vi "XY Dialog.vi"(8 "error in (no error)":errorcluster, 10 "Waveform Graph Data in":T1={"Custom Data"=variant, "EventRegs"={"SystemChange"=refnum, "WorkspaceState"=refnum, "Graph"=refnum, "Wks&Dialog&Periodic"=refnum}, "References"={"X.Scale.Auto"=refnum, "Y.Scale.Auto"=refnum, "X.Scale.Once"=refnum, "Y.Scale.Once"=refnum, "LegendVis"=refnum, "Graph"=refnum}, "Persistent Data"={"Label"="", "Graph Props"={"Plots"=[], "Legend:Number of Rows"=0, "Scale Properties"={"X.Auto"=FALSE, "X.Min"=0.0, "X.Max"=0.0, "X.IgnoreTS"=FALSE, "X.Precision"=0, "X.Label:"="", "X.LabelVis"=FALSE, "X.DefLabel"=FALSE, "Y.Auto"=FALSE, "Y.Min"=0.0, "Y.Max"=0.0, "Y.Format"=0, "Y.Precision:"=0, "Y.Label:"="", "Y.LabelVis"=FALSE, "Y.DefLabel"=FALSE, "X.Format"=0}, "Legend:Visible"=TRUE, "BgColor"=0, "Last Plot Width"=0, "Resize"=FALSE}, "UDP Data"={"Decimation"=0, "UDP Buffer Size"=0, "History Length"=0.0, "Update Rate"=enum."15 Hz", "Channel Paths"=[], "Channel Names"=[]}}, "System"={"To Workspace"=refnum, "From Workspace"=refnum, "NIVS helper"=refnum, "Gtwy"="", "Root"=refnum, "Workspace"=refnum, "SystemStateRefs"={"CustDatRef"=refnum, "EvtRef"=refnum}, "Connected?"=FALSE, "FromDialog"=refnum, "ErrFlag"=FALSE, "New"=FALSE, "ErrState"="", "Save"=FALSE, "Hold"=FALSE, "Periodic"=refnum, "ToDialog"=refnum, "DialogEventReg"=refnum, "UseSavedWidth"=FALSE, "TreeBrowserEventReg"=refnum, "UDPChannelStreamSession"=refnum, "Valid Channels?"=FALSE, "Update Graph"=refnum, "UDP Queue"=refnum, "Graph Update Queue"=refnum}, "GraphData"=[], "UDP Stream Active?"=FALSE} {"Persistent Data"."Graph Props"."Scale Properties"."X.Format" items=["Decimal", "Scientific", "Engineering", "Binary", "Octal", "Hexadecimal", "Relative Time", "Time and Date", "SI", "Automatic"]; "Persistent Data"."Graph Props"."Scale Properties"."Y.Precision:" items=["0", "1", "2", "3", "4", "5", "6", "7"]; "Persistent Data"."Graph Props"."Scale Properties"."Y.Format" items=["Decimal", "Scientific", "Engineering", "Binary", "Octal", "Hexadecimal", "Relative Time", "Time and Date", "SI", "Automatic"]; "Persistent Data"."Graph Props"."Scale Properties"."X.Precision" items=["0", "1", "2", "3", "4", "5", "6", "7"]}) -> ()   [LabVIEW 2013, in "Workspace MultiY Graph.lvlib"]
uses:
  Workspace MultiY Graph.lvlib
  XY Scale Precision.ctl
  XY Scale Format.ctl
  XY Top level workspace graph data.ctl
  <vilib>/NI Veristand/Execution/Workspace/SystemStateRegEventRef.ctl
  <vilib>/NI Veristand/Display Template Support/Display Template Support.llb/enum_Display Template Handler Minimal To Widget Msg.ctl
  XY Dialog Msg to Control.ctl
  XY Dialog Msg Type.ctl
  XY Persistent Data.ctl
  XY Graph Properties.ctl
  XY Plot Properties.ctl
  XY Scale Properties.ctl
  UDP Data.ctl
  Update Rate.ctl
  XY References.ctl
  <vilib>/NI Veristand/Display Template Support/Display Template Support.llb/enum_Display Template Handler Minimal To Workspace.ctl
  NationalInstruments.VeriStand.SystemStorage
  <vilib>/NI Veristand/Execution/Workspace/WorkspaceAPI.ctl
  NationalInstruments.VeriStand.ClientAPI
  <vilib>/NI Veristand/Execution/Workspace/SystemStateEventRef.ctl
  XY Control Msg to Dialog.ctl
  <vilib>/NI Veristand/UI Controls/Tree and Alias Browser/Net Event Data Ref.ctl
  <vilib>/NI Veristand/UI Controls/Tree and Alias Browser/Net Event Data.ctl
  <vilib>/NI Veristand/UI Controls/Tree and Alias Browser/Net Event.ctl
  <vilib>/NI Veristand/Execution/Workspace/UDPChannelStreamSession.ctl
  UDP Queue Data.ctl
  UDP Action State.ctl
  Graph Update Queue Data.ctl
  Graph Update Action State.ctl
  NationalInstruments.VeriStand.SystemStorageUI
  XY Top level dialog data.ctl
  XY Dialog References.ctl
  Dlg Symbol.ctl
  <vilib>/NI Veristand/Execution/Workspace/NI_VS Workspace ExecutionAPI.lvlib
  <vilib>/NI Veristand/UI Controls/Tree and Alias Browser/NI_VS UI Tree Alias Browser.lvlib
  Alert Dialogs.lvlib
panel:
  in  "Cancel":bool
  in  "OK":bool
  in  "Delete":bool
  in  "Tab Control":enum32{"General", "Format & Precision"}(tab)
  in  "Y Channel":i32[](listbox)
  in  "Y Previous":bool
  in  "Y Next":bool
  in  "Tree Browser":refnum<k24>(container)
  in  "X Channel":i32[](listbox)
  in  "X Previous":bool
  in  "X Next":bool
  in  "Resize":bool
  in  "Update Rate:":T11
  in  "History Length:":dbl=0.5 min=0.5 max=3600.0 step=0.5
  in  "UDP Buffer Size:":u32=8192 min=8192 max=65536 step=1
  in  "Decimation:":i32=1 min=1 max=1000000 step=1
  in  "Plot Area Background Color":u32(colorbox)
  in  "Graph Title":string="Waveform Graph"
  in  "X.Format":T9 caption="Format:" items=["Decimal", "Scientific", "Engineering", "Binary", "Octal", "Hexadecimal", "Relative Time", "Time and Date", "SI", "Automatic"]
  in  "X.Min":dbl caption="Minimum:"
  in  "X.Max":dbl caption="Maximum:"
  in  "X.Precision":T8 caption="Precision:" items=["0", "1", "2", "3", "4", "5", "6", "7"]
  in  "Y.Precision":T8 caption="Precision:" items=["0", "1", "2", "3", "4", "5", "6", "7"]
  in  "Y.Format":T9 caption="Format:" items=["Decimal", "Scientific", "Engineering", "Binary", "Octal", "Hexadecimal", "Relative Time", "Time and Date", "SI", "Automatic"]
  in  "X.Label.Default":bool caption="Use Default Label?"
  in  "X.Label.Visible":bool caption="Label Visible?"
  in  "X.Label":string caption="Label:"
  in  "Y.Label.Default":bool caption="Use Default Label?"
  in  "Y.Label.Visible":bool caption="Label Visible?"
  in  "Y.Label":string caption="Label:"
  in  "X.Autoscale":bool caption="Autoscale?"
  in  "Y.Autoscale":bool caption="Autoscale?"
  in  "Y.Min":dbl caption="Minimum:"
  in  "Y.Max":dbl caption="Maximum:"
  # "X Scale"
  # "Y Scale"
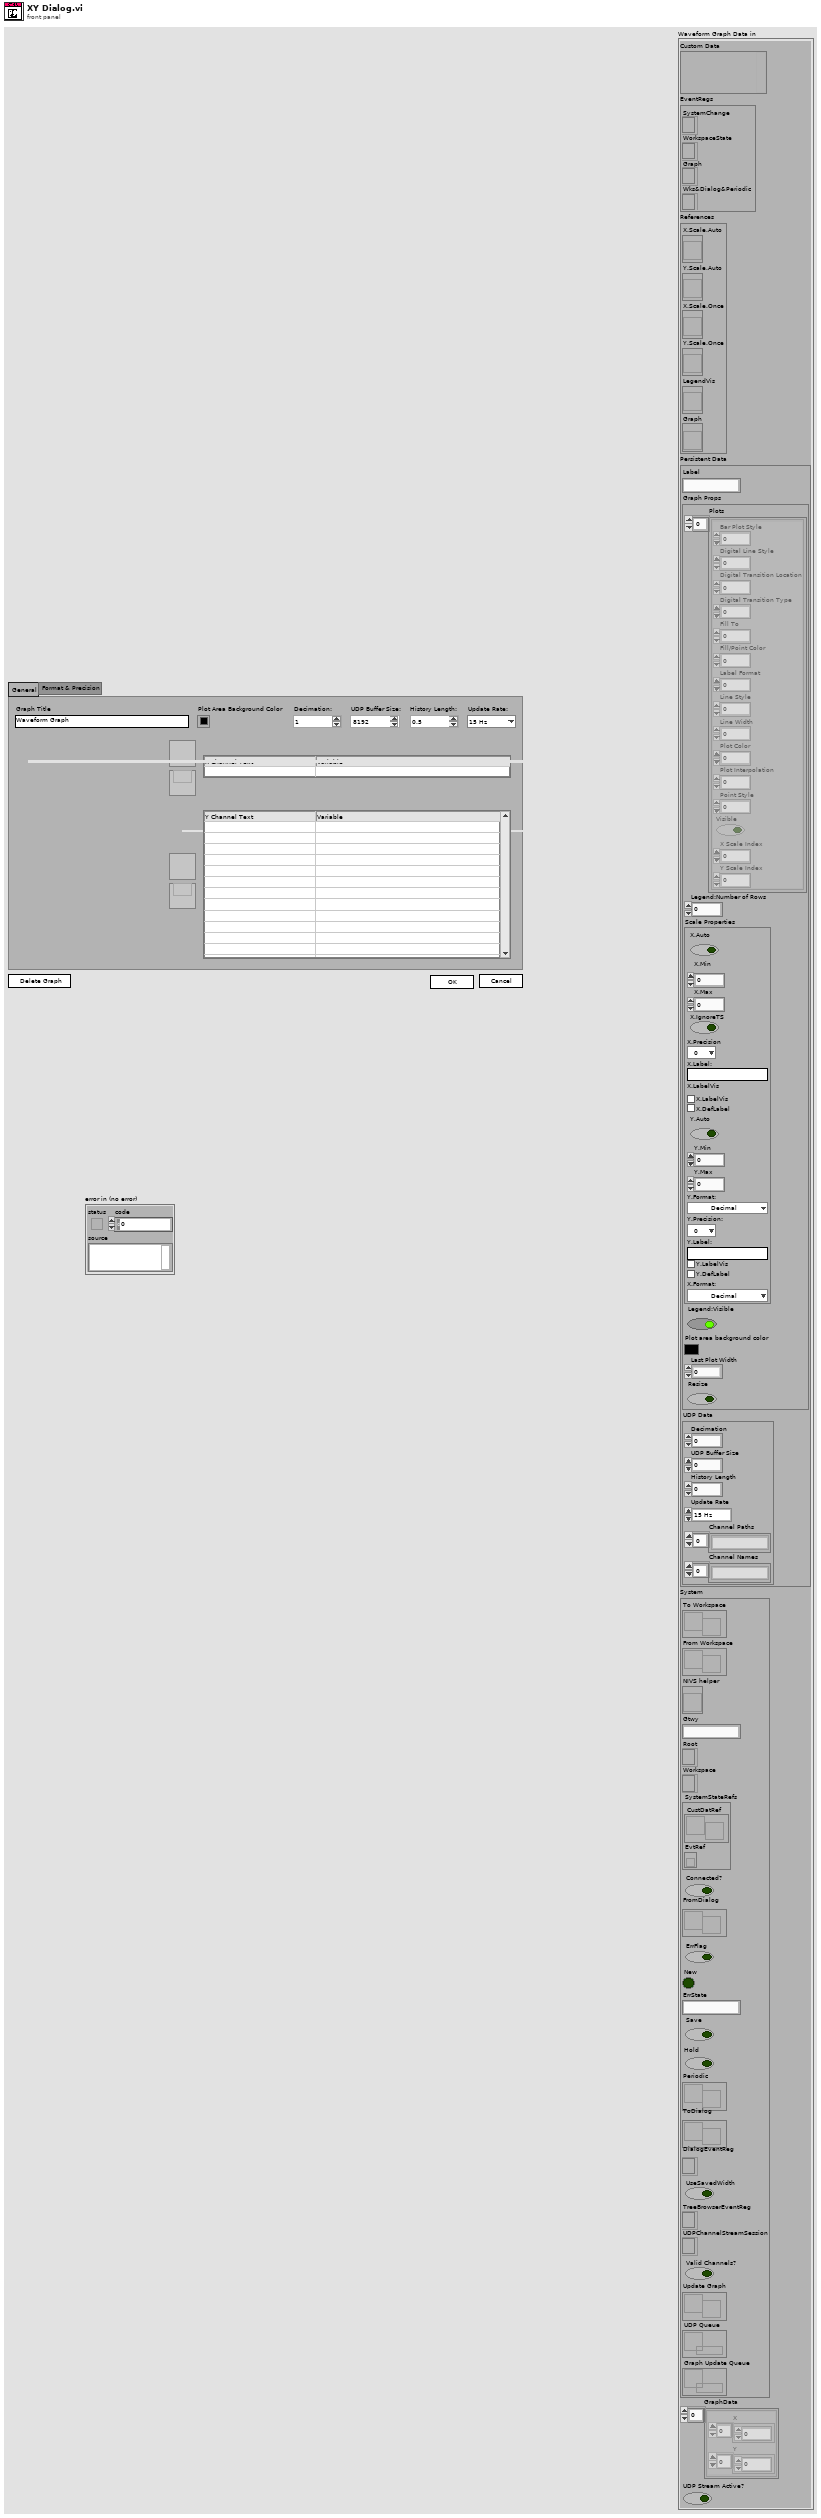
[diagram p1: front panel]
types:
  T1 = typedef "Workspace MultiY Graph.lvlib/XY Top level workspace graph data.ctl" = cluster{"Custom Data":variant, "EventRegs":cluster{"SystemChange":T2, "WorkspaceState":refnum<event-registration>, "Graph":refnum<event-registration>, "Wks&Dialog&Periodic":refnum<event-registration>}, "References":T3, "Persistent Data":T4, "System":cluster{"To Workspace":refnum<user-event>, "From Workspace":refnum<user-event>, "NIVS helper":refnum<vi>, "Gtwy":string, "Root":refnum<k24>, "Workspace":T12, "SystemStateRefs":T13, "Connected?":bool, "FromDialog":refnum<user-event>, "ErrFlag":bool, "New":bool, "ErrState":string, "Save":bool, "Hold":bool, "Periodic":refnum<user-event>, "ToDialog":refnum<user-event>, "DialogEventReg":refnum<event-registration>, "UseSavedWidth":bool, "TreeBrowserEventReg":refnum<event-registration>, "UDPChannelStreamSession":T14, "Valid Channels?":bool, "Update Graph":refnum<user-event>, "UDP Queue":refnum<queue>, "Graph Update Queue":refnum<queue>}, "GraphData":cluster{"X":dbl[], "Y":dbl[]}[], "UDP Stream Active?":bool}
  T2 = typedef "NI_VS Workspace ExecutionAPI.lvlib/SystemStateRegEventRef.ctl" = refnum<event-registration>
  T3 = typedef "Workspace MultiY Graph.lvlib/XY References.ctl" = cluster{"X.Scale.Auto":refnum<vi>, "Y.Scale.Auto":refnum<vi>, "X.Scale.Once":refnum<vi>, "Y.Scale.Once":refnum<vi>, "LegendVis":refnum<vi>, "Graph":refnum<vi>}
  T4 = typedef "Workspace MultiY Graph.lvlib/XY Persistent Data.ctl" = cluster{"Label":string, "Graph Props":T5, "UDP Data":T10}
  T5 = typedef "Workspace MultiY Graph.lvlib/XY Graph Properties.ctl" = cluster{"Plots":T6[], "Legend:Number of Rows":u32, "Scale Properties":T7, "Legend:Visible":bool, "BgColor":u32, "Last Plot Width":u32, "Resize":bool}
  T6 = typedef "Workspace MultiY Graph.lvlib/XY Plot Properties.ctl" = cluster{"Bar Plot Style":u8, "Digital Line Style":u8, "Digital Transition Location":u8, "Digital Transition Type":u8, "Fill To":i16, "Fill/Point Color":u32, "Label Format":u8, "Line Style":u8, "Line Width":u8, "Plot Color":u32, "Plot Interpolation":u8, "Point Style":u8, "Visible":bool, "X Scale Index":u32, "Y Scale Index":u32}
  T7 = typedef "Workspace MultiY Graph.lvlib/XY Scale Properties.ctl" = cluster{"X.Auto":bool, "X.Min":dbl, "X.Max":dbl, "X.IgnoreTS":bool, "X.Precision":T8, "X.Label:":string, "X.LabelVis":bool, "X.DefLabel":bool, "Y.Auto":bool, "Y.Min":dbl, "Y.Max":dbl, "Y.Format":T9, "Y.Precision:":T8, "Y.Label:":string, "Y.LabelVis":bool, "Y.DefLabel":bool, "X.Format":T9}
  T8 = typedef "Workspace MultiY Graph.lvlib/XY Scale Precision.ctl" = u8
  T9 = typedef "Workspace MultiY Graph.lvlib/XY Scale Format.ctl" = u8
  T10 = typedef "Workspace MultiY Graph.lvlib/UDP Data.ctl" = cluster{"Decimation":i32, "UDP Buffer Size":u32, "History Length":dbl, "Update Rate":T11, "Channel Paths":string[], "Channel Names":string[]}
  T11 = typedef "Workspace MultiY Graph.lvlib/Update Rate.ctl" = enum8{"15 Hz", "10 Hz", "5 Hz", "4 Hz", "3 Hz", "2 Hz", "1 Hz", "0.5 Hz"}
  T12 = typedef "NI_VS Workspace ExecutionAPI.lvlib/WorkspaceAPI.ctl" = refnum<k24>
  T13 = typedef "NI_VS Workspace ExecutionAPI.lvlib/SystemStateEventRef.ctl" = cluster{"CustDatRef":refnum<user-event>, "EvtRef":refnum<k27>}
  T14 = typedef "NI_VS Workspace ExecutionAPI.lvlib/UDPChannelStreamSession.ctl" = refnum<k24>
  T15 = typedef "Workspace MultiY Graph.lvlib/XY Top level dialog data.ctl" = cluster{"GraphData":T1, "References":T16, "Tree Selected Paths":string[][], "SelectedIdx":i32, "dts":dbl[], "X Selected Paths":string[][], "Y Selected Paths":string[][]}
  T16 = typedef "Workspace MultiY Graph.lvlib/XY Dialog References.ctl" = cluster{"BgColor":refnum<vi>, "Title":refnum<vi>, "Waveforms":refnum<vi>, "PointsPerPixel":refnum<vi>, "Low":refnum<vi>, "High":refnum<vi>, "History":refnum<vi>, "N":refnum<vi>, "M":refnum<vi>, "IgnTimeStamp":refnum<vi>, "X.Precision":refnum<vi>, "X.Label":refnum<vi>, "X.Label.Default":refnum<vi>, "X.Label.Visible":refnum<vi>, "X.Autoscale":refnum<vi>, "X.Max":refnum<vi>, "X.Min":refnum<vi>, "Y.Format":refnum<vi>, "Y.Precision":refnum<vi>, "Y.Label":refnum<vi>, "Y.Label.Default":refnum<vi>, "Y.Label.Visible":refnum<vi>, "Y.Autoscale":refnum<vi>, "Y.Max":refnum<vi>, "Y.Min":refnum<vi>, "rate":refnum<vi>, "path":refnum<vi>, "Alias TreeBrowser":refnum<vi>, "Y Channel Listbox":refnum<vi>, "X Channel Listbox":refnum<vi>, "X.Format":refnum<vi>, "X Next":refnum<vi>, "Y Next":refnum<vi>, "X Previous":refnum<vi>, "Y Previous":refnum<vi>, "Decimation":refnum<vi>, "History Length":refnum<vi>, "UDP Buffer Size":refnum<vi>}
  T17 = typedef "Workspace MultiY Graph.lvlib/Alert Dialogs.lvlib/Dlg Symbol.ctl" = enum16{"Information", "Help", "Warning", "Error"}
  T18 = enum8{"Enabled", "Disabled", "Disabled and Grayed Out"}
  T19 = typedef "Workspace MultiY Graph.lvlib/XY Dialog Msg Type.ctl" = enum16{"Update", "Delete"}
  T20 = typedef "Workspace MultiY Graph.lvlib/XY Dialog Msg to Control.ctl" = cluster{"DialogMsgType":T19, "Persistent Data":T4}
  T21 = cluster{"TreeBrowserEventReg":refnum<event-registration>, "DialogEventReg":refnum<event-registration>}
  T22 = typedef "Workspace MultiY Graph.lvlib/XY Control Msg to Dialog.ctl" = enum16{"Stop", "Connecting", "Disconnecting"}
  T23 = typedef "Workspace MultiY Graph.lvlib/Alert Dialogs.lvlib/Dlg Button.ctl" = enum16{"Left Button", "Center Button", "Right Button", "Window Close"}
  T24 = typedef "NI_VS UI Tree Alias Browser.lvlib/Net Event.ctl" = enum16{"SelectedItem", "DblClick"}
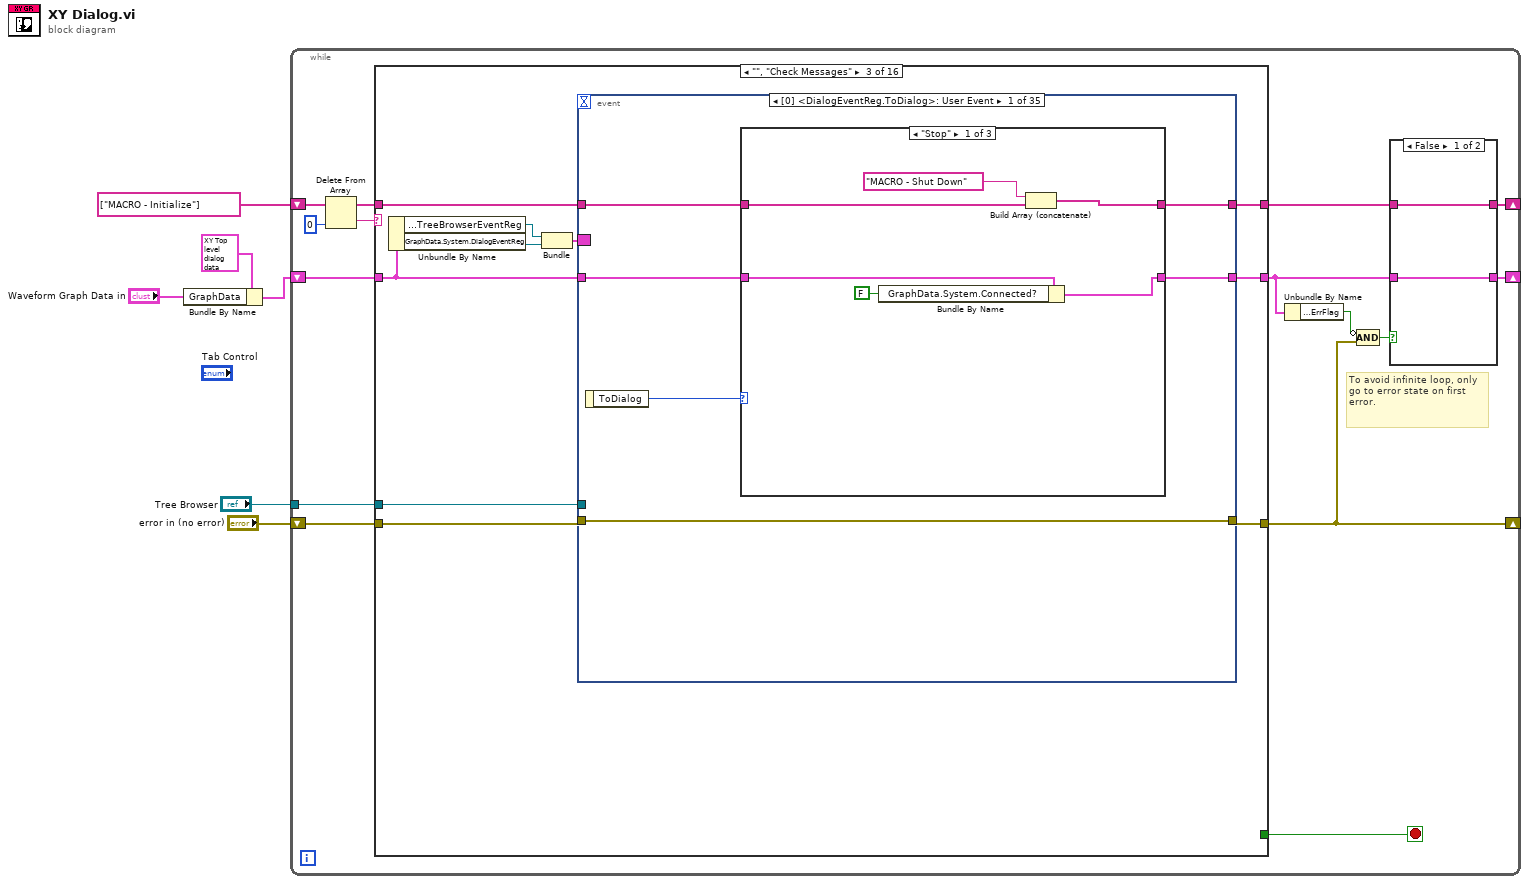
[diagram p0: block diagram]
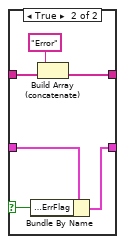
[diagram p2: hidden frame]
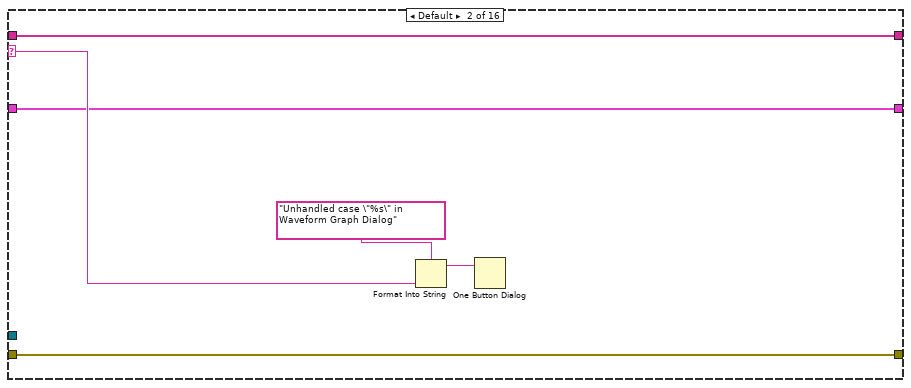
[diagram p4: hidden frame]
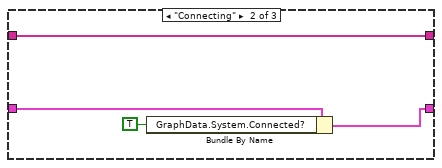
[diagram p5: hidden frame]
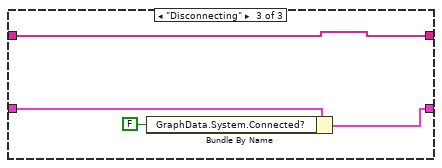
[diagram p6: hidden frame]
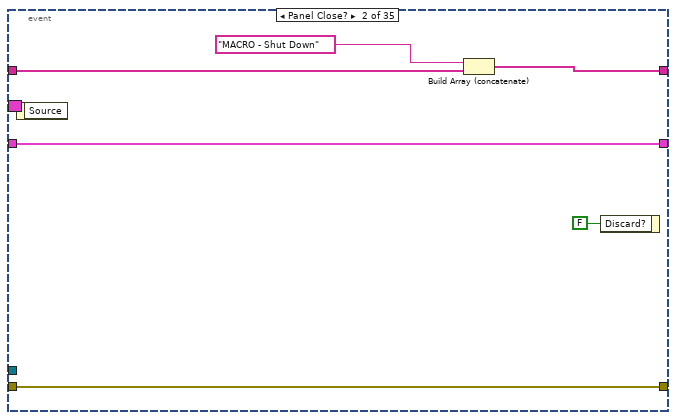
[diagram p7: hidden frame]
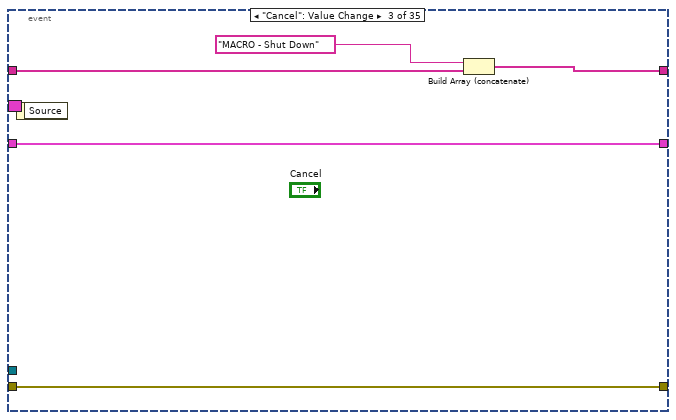
[diagram p8: hidden frame]
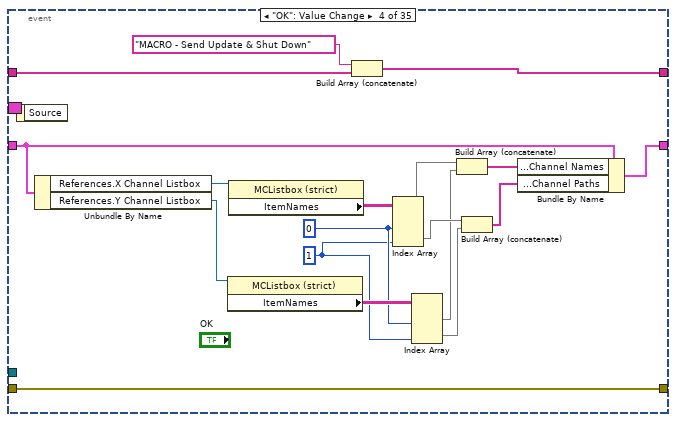
[diagram p9: hidden frame]
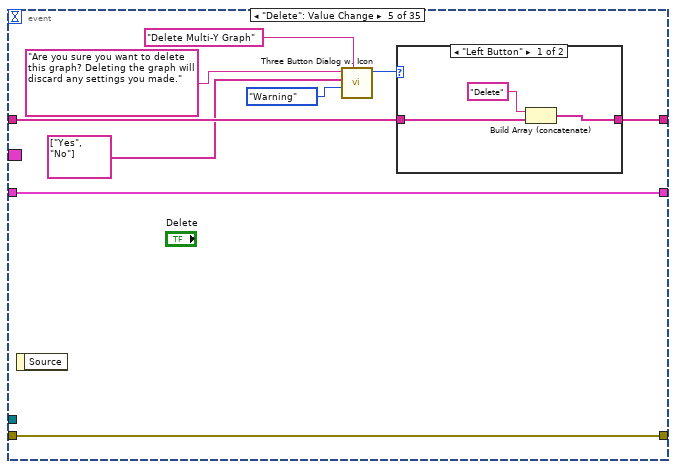
[diagram p10: hidden frame]
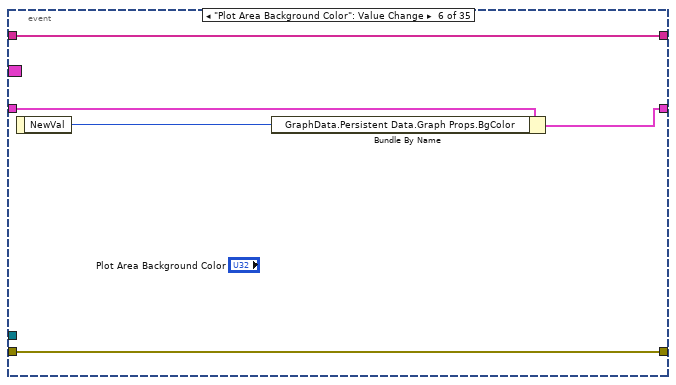
[diagram p12: hidden frame]
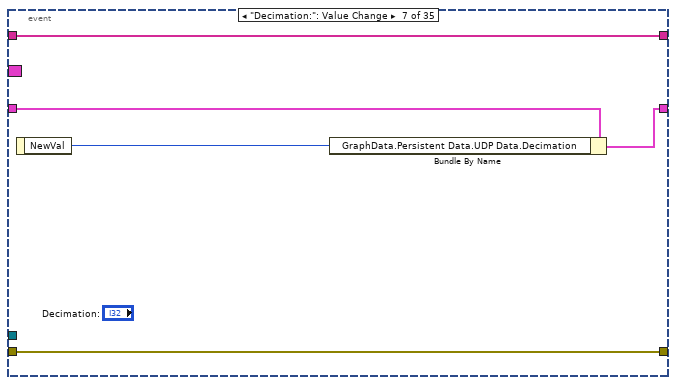
[diagram p13: hidden frame]
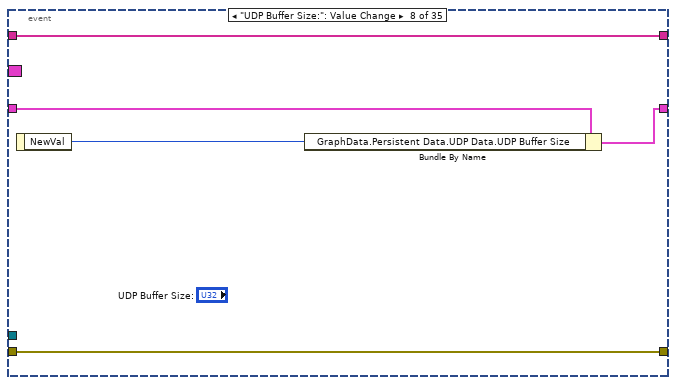
[diagram p14: hidden frame]
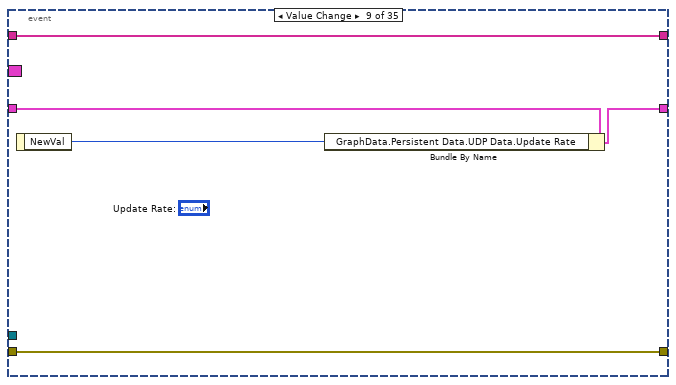
[diagram p15: hidden frame]
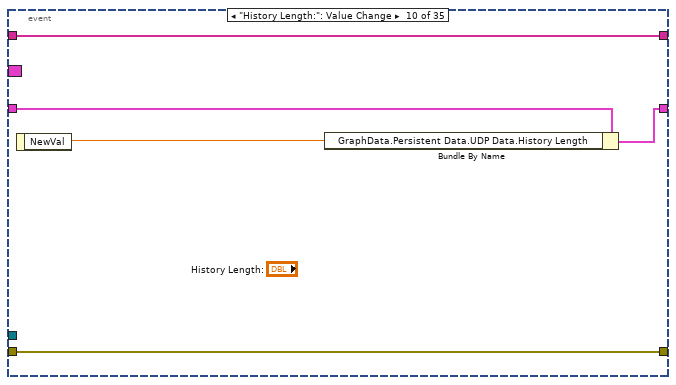
[diagram p16: hidden frame]
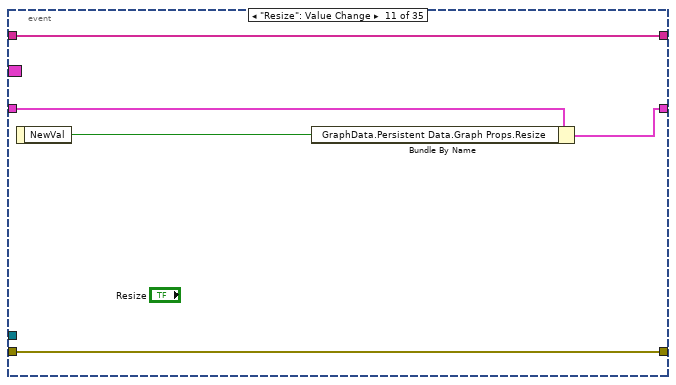
[diagram p17: hidden frame]
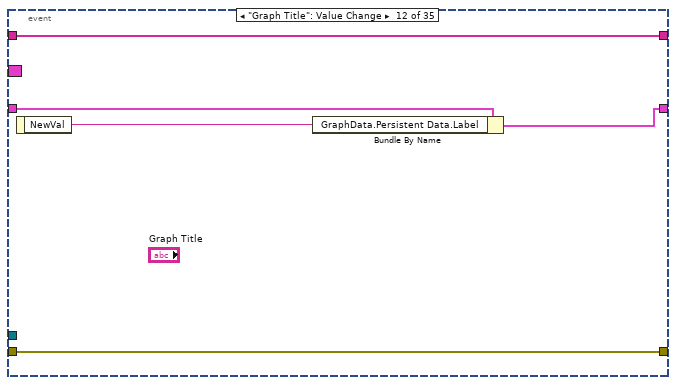
[diagram p18: hidden frame]
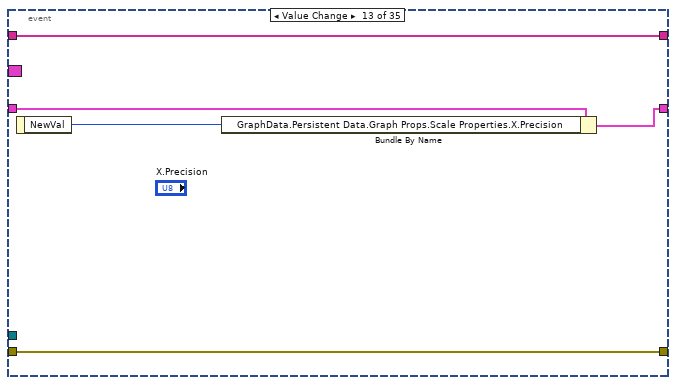
[diagram p19: hidden frame]
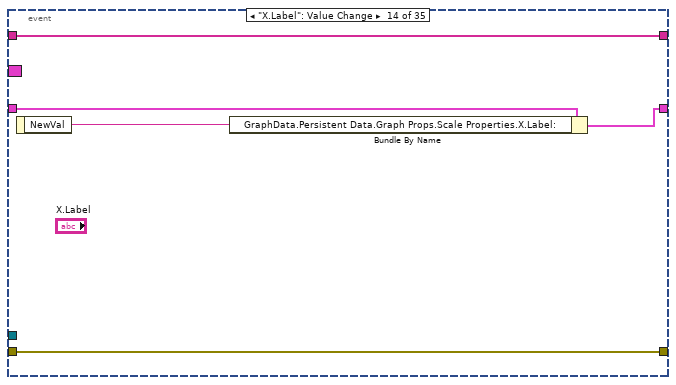
[diagram p20: hidden frame]
diagram:
  n1 = Bundle By Name(cluster=T15 {"GraphData"={"Custom Data"=variant, "EventRegs"={"SystemChange"=refnum, "WorkspaceState"=refnum, "Graph"=refnum, "Wks&Dialog&Periodic"=refnum}, "References"={"X.Scale.Auto"=refnum, "Y.Scale.Auto"=refnum, "X.Scale.Once"=refnum, "Y.Scale.Once"=refnum, "LegendVis"=refnum, "Graph"=refnum}, "Persistent Data"={"Label"="", "Graph Props"={"Plots"=[], "Legend:Number of Rows"=0, "Scale Properties"={"X.Auto"=FALSE, "X.Min"=0.0, "X.Max"=0.0, "X.IgnoreTS"=FALSE, "X.Precision"=0, "X.Label:"="", "X.LabelVis"=FALSE, "X.DefLabel"=FALSE, "Y.Auto"=FALSE, "Y.Min"=0.0, "Y.Max"=0.0, "Y.Format"=0, "Y.Precision:"=0, "Y.Label:"="", "Y.LabelVis"=FALSE, "Y.DefLabel"=FALSE, "X.Format"=0}, "Legend:Visible"=FALSE, "BgColor"=0, "Last Plot Width"=0, "Resize"=FALSE}, "UDP Data"={"Decimation"=0, "UDP Buffer Size"=0, "History Length"=0.0, "Update Rate"=enum."15 Hz", "Channel Paths"=[], "Channel Names"=[]}}, "System"={"To Workspace"=refnum, "From Workspace"=refnum, "NIVS helper"=refnum, "Gtwy"="", "Root"=refnum, "Workspace"=refnum, "SystemStateRefs"={"CustDatRef"=refnum, "EvtRef"=refnum}, "Connected?"=FALSE, "FromDialog"=refnum, "ErrFlag"=FALSE, "New"=FALSE, "ErrState"="", "Save"=FALSE, "Hold"=FALSE, "Periodic"=refnum, "ToDialog"=refnum, "DialogEventReg"=refnum, "UseSavedWidth"=FALSE, "TreeBrowserEventReg"=refnum, "UDPChannelStreamSession"=refnum, "Valid Channels?"=FALSE, "Update Graph"=refnum, "UDP Queue"=refnum, "Graph Update Queue"=refnum}, "GraphData"=[], "UDP Stream Active?"=FALSE}, "References"={"BgColor"=refnum, "Title"=refnum, "Waveforms"=refnum, "PointsPerPixel"=refnum, "Low"=refnum, "High"=refnum, "History"=refnum, "N"=refnum, "M"=refnum, "IgnTimeStamp"=refnum, "X.Precision"=refnum, "X.Label"=refnum, "X.Label.Default"=refnum, "X.Label.Visible"=refnum, "X.Autoscale"=refnum, "X.Max"=refnum, "X.Min"=refnum, "Y.Format"=refnum, "Y.Precision"=refnum, "Y.Label"=refnum, "Y.Label.Default"=refnum, "Y.Label.Visible"=refnum, "Y.Autoscale"=refnum, "Y.Max"=refnum, "Y.Min"=refnum, "rate"=refnum, "path"=refnum, "Alias TreeBrowser"=refnum, "Y Channel Listbox"=refnum, "X Channel Listbox"=refnum, "X.Format"=refnum, "X Next"=refnum, "Y Next"=refnum, "X Previous"=refnum, "Y Previous"=refnum, "Decimation"=refnum, "History Length"=refnum, "UDP Buffer Size"=refnum}, "Tree Selected Paths"=[], "SelectedIdx"=0, "dts"=[], "X Selected Paths"=[], "Y Selected Paths"=[]} ("Dialog Data"), "GraphData"="Waveform Graph Data in") -> (w5:T15)
  n2 = while {
    shift-right: [w16] -> _
    shift-left: string[] ["MACRO - Initialize"] -> [w21]
    shift-right: [w8] -> _
    shift-left: "error in (no error)" -> [w15]
    shift-right: [w12] -> _
    shift-left: w5 -> [w17]
    tunnel: "Tree Browser" -> [w7]
    stop <- w19 stop-if-true
    # "To avoid infinite loop, only go to error state on first error."
    n3 = Delete From Array(array=w21, index=0) -> (deleted portion=w14:string, array with subset deleted=w20:string[])  [unwired: 1 in]
    n4 = case shown="\"\", \"Check Messages\"" w14 {
      selector: w14 -> [_ w37 _ _ _ _ _ _ _ _ _ _ _ _ _ _]
      tunnel: [w30 w33 w48 string[] ["MACRO - Shut Down"] w353 w365 w367 w371 w375 w379 w385 w389 w393 w425 w441 w450] -> w18
      tunnel: w20 -> [w30 w33 w47 _ w353 w366 w367 w371 w375 w380 w386 w390 w393 w425 w441 w450]
      tunnel: [_ _ _ _ _ _ _ TRUE _ _ _ _ _ _ _ _] -> w19
      tunnel: w15 -> [w32 w35 w45 w347 w355 w362 w369 w373 w377 w382 w387 w392 w395 w424 w440 w448]
      tunnel: [w32 w35 w44 errorcluster {"status"=FALSE, "code"=0, "source"=""} ("error constant") w352 w359 w369 w373 w377 w382 w387 w392 w395 w424 w439 w444] -> w8
      tunnel: w17 -> [w31 w34 w43 w344 w356 w363 w368 w372 w376 w378 w384 w391 w394 w427 w436 w449]
      tunnel: [w31 w34 w46 w344 w356 w363 w368 w372 w376 w378 w384 w391 w394 w426 w434 w449] -> w11
      tunnel: w7 -> [_ _ w39 _ _ _ _ _ _ _ _ _ _ _ w433 _]
      frame "<------------------ System ------------------>" {
      }
      frame Default {
        n5 = Format Into String(format string="Unhandled case \"%s\" in Waveform Graph Dialog", w37) -> (resulting string=w38:string)  [unwired: 2 in, 1 out]
        n6 = One Button Dialog(message=w38) -> ()  [unwired: 1 in, 1 out]
      }
      frame "", "Check Messages" {
        n7 = Unbundle By Name(w43) -> ("GraphData.System.TreeBrowserEventReg"=w42:refnum<event-registration>, "GraphData.System.DialogEventReg"=w41:refnum<event-registration>)
        n8 = Bundle("TreeBrowserEventReg"=w42, "DialogEventReg"=w41) -> (w40:T21)  [unwired: 1 in]
        n9 = event shown="[0] <DialogEventReg.ToDialog>: User Event" {
          selector: w40 -> [_ _ _ _ _ _ _ _ _ _ _ _ _ _ _ _ _ _ _ _ _ _ _ _ _ _ _ _ _ _ _ _ _ _ _]
          dyn-events: _ -> [_ _ _ _ _ _ _ _ _ _ _ _ _ _ _ _ _ _ _ _ _ _ _ _ _ _ _ _ _ _ _ _ _ _ _]
          timeout: _ -> [_ _ _ _ _ _ _ _ _ _ _ _ _ _ _ _ _ _ _ _ _ _ _ _ _ _ _ _ _ _ _ _ _ _ _]
          tunnel: [w51 w70 w76 w95 w103 w115 w120 w125 w130 w135 w140 w145 w150 w155 w160 w165 w181 w193 w203 w209 w220 w236 w246 w251 w260 w271 w278 w283 w288 w293 w309 w318 w323 w333 w343] -> w48
          tunnel: w47 -> [w52 w74 w79 w97 w106 w115 w120 w125 w130 w135 w140 w145 w150 w155 w160 w165 w181 w193 w203 w209 w220 w236 w246 w251 w260 w271 w278 w283 w288 w293 w309 w318 w323 w333 w343]
          tunnel: [w50 w73 w78 w90 w105 w112 w117 w122 w127 w132 w137 w142 w147 w152 w157 w162 w180 w190 w202 w208 w219 w235 w243 w248 w259 w270 w277 w280 w285 w290 w308 w315 w320 w324 w342] -> w46
          tunnel: w43 -> [w49 w73 w78 w91 w105 w114 w118 w123 w128 w133 w138 w144 w149 w154 w159 w164 w179 w188 w202 w208 w219 w235 w245 w250 w255 w266 w276 w282 w287 w292 w307 w317 w322 w324 w342]
          tunnel: w45 -> [w54 w72 w77 w96 w104 w113 w119 w124 w129 w134 w139 w143 w148 w153 w158 w163 w176 w192 w198 w205 w215 w232 w244 w249 w253 w264 w274 w281 w286 w291 w304 w316 w321 w331 w340]
          tunnel: [w54 w72 w77 w96 w104 w113 w119 w124 w129 w134 w139 w143 w148 w153 w158 w163 w171 w191 w195 w207 w211 w229 w244 w249 w256 w267 w274 w281 w286 w291 w301 w316 w321 w330 w339] -> w44
          tunnel: w39 -> [_ _ _ _ _ _ _ _ _ _ _ _ _ _ _ _ _ w189 _ _ _ _ _ _ _ _ _ _ _ _ _ _ _ _ _]
          event User Event {
            n10 = event-data() -> ("ToDialog"=w53:T22)  [unwired: 1 in]
            n11 = case shown="\"Stop\"" w53 {
              tunnel: w52 -> [w59 w61 w65]
              tunnel: [w58 w61 w65] -> w51
              tunnel: [w56 w63 w67] -> w50
              tunnel: w49 -> [w57 w64 w68]
              frame "Stop" {
                n12 = Bundle By Name(cluster=w57, "GraphData.System.Connected?"=FALSE) -> (w56:T15)
                n13 = Build Array (concatenate)("MACRO - Shut Down", w59) -> (w58:string[])
              }
              frame "Connecting" {
                n14 = Bundle By Name(cluster=w64, "GraphData.System.Connected?"=TRUE) -> (w63:T15)
              }
              frame "Disconnecting" {
                n15 = Bundle By Name(cluster=w68, "GraphData.System.Connected?"=FALSE) -> (w67:T15)
              }
            }
          }
          event Panel Close? {
            n16 = event-data() -> ()  [unwired: 1 in, 1 out]
            n17 = Build Array (concatenate)("MACRO - Shut Down", w74) -> (w70:string[])
            n18 = event-data("Discard?"=FALSE) -> ()  [unwired: 1 in, 1 out]
          }
          event "Cancel": Value Change {
            n19 = event-data() -> ()  [unwired: 1 in, 1 out]
            n20 = Build Array (concatenate)("MACRO - Shut Down", w79) -> (w76:string[])
          }
          event "OK": Value Change {
            w80 = 1 ("index (row)")
            w81 = 0 ("index (row)")
            n21 = event-data() -> ()  [unwired: 1 in, 1 out]
            n22 = Unbundle By Name(w91) -> ("References.X Channel Listbox"=w93:refnum<vi>, "References.Y Channel Listbox"=w92:refnum<vi>)
            n23 = property class="MCListbox (strict)"(reference=w92) -> ("ItemNames"=w88:string[][])  [unwired: 1 in, 2 out]
            n24 = property class="MCListbox (strict)"(reference=w93) -> ("ItemNames"=w89:string[][])  [unwired: 1 in, 2 out]
            n25 = Build Array (concatenate)("MACRO - Send Update & Shut Down", w97) -> (w95:string[])
            n26 = Index Array(array=w89, index (col) #1=w81, index (col) #2=w80) -> (element #1=w84:string[], element #2=w85:string[])  [unwired: 2 in]
            n27 = Index Array(array=w88, index (col) #1=w81, index (col) #2=w80) -> (element #1=w83:string[], element #2=w86:string[])  [unwired: 2 in]
            n28 = Build Array (concatenate)(w84, w83) -> (w82:string[])
            n29 = Build Array (concatenate)(w85, w86) -> (w87:string[])
            n30 = Bundle By Name(cluster=w91, "GraphData.Persistent Data.UDP Data.Channel Names"=w82, "GraphData.Persistent Data.UDP Data.Channel Paths"=w87) -> (w90:T15)
          }
          event "Delete": Value Change {
            n31 = event-data() -> ()  [unwired: 1 in, 1 out]
            n32 = call "Three Button Dialog w. Icon.vi"("Window Title (\"\")"="Delete Multi-Y Graph" ("Window Title (\"\")"), "Symbol"=Dlg_Symbol."Warning", "Button Strings"=string[] ["Yes", "No"], "Message"="Are you sure you want to delete this graph? Deleting the graph will discard any settings you made.") -> ("Which Button?"=w102:T23)  [unwired: 7 in]
            n33 = case shown="\"Left Button\"" w102 {
              tunnel: w106 -> [w109 w110]
              tunnel: [w108 w110] -> w103
              frame "Left Button" {
                n34 = Build Array (concatenate)("Delete", w109) -> (w108:string[])
              }
              frame Default {
              }
            }
          }
          event "Plot Area Background Color": Value Change {
            n35 = event-data() -> ("NewVal"=w111:u32)  [unwired: 1 in]
            n36 = Bundle By Name(cluster=w114, "GraphData.Persistent Data.Graph Props.BgColor"=w111) -> (w112:T15)
          }
          event "Decimation:": Value Change {
            n37 = event-data() -> ("NewVal"=w116:i32)  [unwired: 1 in]
            n38 = Bundle By Name(cluster=w118, "GraphData.Persistent Data.UDP Data.Decimation"=w116) -> (w117:T15)
          }
          event "UDP Buffer Size:": Value Change {
            n39 = event-data() -> ("NewVal"=w121:u32)  [unwired: 1 in]
            n40 = Bundle By Name(cluster=w123, "GraphData.Persistent Data.UDP Data.UDP Buffer Size"=w121) -> (w122:T15)
          }
          event Value Change {
            n41 = event-data() -> ("NewVal"=w126:T11)  [unwired: 1 in]
            n42 = Bundle By Name(cluster=w128, "GraphData.Persistent Data.UDP Data.Update Rate"=w126) -> (w127:T15)
          }
          event "History Length:": Value Change {
            n43 = event-data() -> ("NewVal"=w131:dbl)  [unwired: 1 in]
            n44 = Bundle By Name(cluster=w133, "GraphData.Persistent Data.UDP Data.History Length"=w131) -> (w132:T15)
          }
          event "Resize": Value Change {
            n45 = event-data() -> ("NewVal"=w136:bool)  [unwired: 1 in]
            n46 = Bundle By Name(cluster=w138, "GraphData.Persistent Data.Graph Props.Resize"=w136) -> (w137:T15)
          }
          event "Graph Title": Value Change {
            n47 = event-data() -> ("NewVal"=w141:string)  [unwired: 1 in]
            n48 = Bundle By Name(cluster=w144, "GraphData.Persistent Data.Label"=w141) -> (w142:T15)
          }
          event Value Change {
            n49 = event-data() -> ("NewVal"=w146:T8)  [unwired: 1 in]
            n50 = Bundle By Name(cluster=w149, "GraphData.Persistent Data.Graph Props.Scale Properties.X.Precision"=w146) -> (w147:T15)
          }
          event "X.Label": Value Change {
            n51 = event-data() -> ("NewVal"=w151:string)  [unwired: 1 in]
            n52 = Bundle By Name(cluster=w154, "GraphData.Persistent Data.Graph Props.Scale Properties.X.Label:"=w151) -> (w152:T15)
          }
          event "X.Label.Default": Value Change {
            n53 = event-data() -> ("NewVal"=w156:bool)  [unwired: 1 in]
            n54 = Bundle By Name(cluster=w159, "GraphData.Persistent Data.Graph Props.Scale Properties.X.DefLabel"=w156) -> (w157:T15)
          }
          event "X.Label.Visible": Value Change {
            n55 = event-data() -> ("NewVal"=w161:bool)  [unwired: 1 in]
            n56 = Bundle By Name(cluster=w164, "GraphData.Persistent Data.Graph Props.Scale Properties.X.LabelVis"=w161) -> (w162:T15)
          }
          event "X.Autoscale": Value Change {
            n57 = event-data() -> ("NewVal"=w175:bool)  [unwired: 1 in]
            n58 = Unbundle By Name(w179) -> ("GraphData.References.Graph"=w173:refnum<vi>, "References.X.Max"=w178:refnum<vi>, "References.X.Min"=w177:refnum<vi>)
            n59 = Bundle By Name(cluster=w179, "GraphData.Persistent Data.Graph Props.Scale Properties.X.Auto"=w175) -> (w180:T15)
            n60 = Not(x=w175) -> (.not. x?=w174:bool)
            n61 = Build Array(w178, w177) -> (w172:refnum<vi>[])
            n62 = call "XY Set Control Enable State.vi"("error in (no error)"=w176, "Enabled?"=w174, "Controls"=w172) -> ("error out"=w170:errorcluster)  [unwired: 8 in]
            n63 = property class="XYGraph (strict)"(reference=w173, error in=w170) -> (error out=w169:errorcluster, "XScale.Maximum"=w168:dbl, "XScale.Minimum"=w167:dbl)  [unwired: 1 out]
            n64 = Build Array(w168, w167) -> (w166:dbl[])
            n65 = for {
              shift-right: [w184] -> w171
              shift-left: w169 -> [w185]
              tunnel: w172 -> [w183] mode=indexing
              tunnel: w166 -> [w182] mode=indexing
              n66 = property class="DigNum (strict)"(reference=w183, error in=w185, "Val(Sgnl)"=w182) -> (error out=w184:errorcluster)  [unwired: 1 out]
            }
          }
          event User Event {
            n67 = event-data() -> ("Data"=w187:variant, "Type"=w186:T24)  [unwired: 1 in, 3 out]
            n68 = call "XY Dialog - Update Selected Paths.vi"("Data"=w187, "error in (no error)"=w192, "Type"=w186, "Tree Browser Refnun"=w189, "Dialog Data in"=w188) -> ("error out"=w191:errorcluster, "Dialog Data out"=w190:T15)  [unwired: 5 in]
          }
          event "X Next": Value Change {
            n69 = event-data() -> ()  [unwired: 1 in, 1 out]
            n70 = Unbundle By Name(w202) -> ("References.X Channel Listbox"=w201:refnum<vi>, "Tree Selected Paths"=w200:string[][])
            n71 = Index Array(array=w200, index (row)=0) -> (element=w197:string[])  [unwired: 1 in]
            n72 = Build Array(w197) -> (w196:string[][])
            n73 = property class="MCListbox (strict)"(reference=w201, error in=w198, "ItemNames"=w196, "Val(Sgnl)"=i32[] [] ("Value (Signaling)")) -> (error out=w195:errorcluster)  [unwired: 1 out]
          }
          event "Y Next": Value Change {
            n74 = event-data() -> ()  [unwired: 1 in, 1 out]
            n75 = Unbundle By Name(w208) -> ("References.Y Channel Listbox"=w206:refnum<vi>, "Tree Selected Paths"=w204:string[][])
            n76 = call "XY Dialog - Update Y Plots.vi"("error in (no error)"=w205, "Tree Selected Paths"=w204, "Y Channel Listbox"=w206) -> ("error out"=w207:errorcluster)  [unwired: 8 in]
          }
          event "X Previous": Value Change {
            n77 = event-data() -> ()  [unwired: 1 in, 1 out]
            n78 = Unbundle By Name(w219) -> ("References.X Channel Listbox"=w218:refnum<vi>)
            n79 = property class="MCListbox (strict)"(reference=w218, error in=w215) -> (reference out=w216:refnum<vi>, error out=w214:errorcluster, "ItemNames"=w217:string[][], "Value"=w210:i32[])
            n80 = for {
              tunnel: w210 -> [w222] mode=indexing
              shift-right: [w224] -> w213
              shift-left: w217 -> [w225]
              i -> [w223]
              n81 = Subtract(x=w222, y=w223) -> (x-y=w221:i32)
              n82 = Delete From Array(array=w225, index (row)=w221) -> (array with subset deleted=w224:string[][])  [unwired: 2 in, 1 out]
            }
            n83 = property class="MCListbox (strict)"(reference=w216, error in=w214, "ItemNames"=w213, "Val(Sgnl)"=i32[] [] ("Value (Signaling)")) -> (error out=w211:errorcluster)  [unwired: 1 out]
          }
          event "Y Previous": Value Change {
            n84 = event-data() -> ()  [unwired: 1 in, 1 out]
            n85 = Unbundle By Name(w235) -> ("References.Y Channel Listbox"=w234:refnum<vi>)
            n86 = property class="MCListbox (strict)"(reference=w234, error in=w232) -> (reference out=w233:refnum<vi>, error out=w231:errorcluster, "ItemNames"=w227:string[][], "Value"=w226:i32[])
            n87 = for {
              shift-right: [w237] -> w230
              shift-left: w227 -> [w241]
              tunnel: w226 -> [w239] mode=indexing
              i -> [w240]
              n88 = Subtract(x=w239, y=w240) -> (x-y=w238:i32)
              n89 = Delete From Array(array=w241, index (row)=w238) -> (array with subset deleted=w237:string[][])  [unwired: 2 in, 1 out]
            }
            n90 = property class="MCListbox (strict)"(reference=w233, error in=w231, "ItemNames"=w230, "Val(Sgnl)"=i32[] [] ("Value (Signaling)")) -> (error out=w229:errorcluster)  [unwired: 1 out]
          }
          event "X.Min": Value Change {
            n91 = event-data() -> ("NewVal"=w242:dbl)  [unwired: 1 in]
            n92 = Bundle By Name(cluster=w245, "GraphData.Persistent Data.Graph Props.Scale Properties.X.Min"=w242) -> (w243:T15)
          }
          event "X.Max": Value Change {
            n93 = event-data() -> ("NewVal"=w247:dbl)  [unwired: 1 in]
            n94 = Bundle By Name(cluster=w250, "GraphData.Persistent Data.Graph Props.Scale Properties.X.Max"=w247) -> (w248:T15)
          }
          event Value Change {
            n95 = event-data() -> ("NewVal"=w254:T9)  [unwired: 1 in]
            n96 = case shown="Default" w254 {
              tunnel: [TRUE FALSE] -> w252
              frame Default {
              }
              frame 9 {
                # "Auto formatting"
              }
            }
            n97 = Unbundle By Name(w255) -> ("References.Y.Precision"=w258:refnum<vi>)
            n98 = Bundle By Name(cluster=w255, "GraphData.Persistent Data.Graph Props.Scale Properties.Y.Format"=w254) -> (w259:T15)
            n99 = Build Array(w258) -> (w257:refnum<vi>[])
            n100 = call "XY Set Control Enable State.vi"("error in (no error)"=w253, "Enabled?"=w252, "Controls"=w257) -> ("error out"=w256:errorcluster)  [unwired: 8 in]
          }
          event Value Change {
            n101 = event-data() -> ("NewVal"=w265:T9)  [unwired: 1 in]
            n102 = case shown="9" w265 {
              tunnel: [TRUE FALSE] -> w263
              frame Default {
              }
              frame 9 {
                # "Auto formatting"
              }
            }
            n103 = Unbundle By Name(w266) -> ("References.X.Precision"=w269:refnum<vi>)
            n104 = Bundle By Name(cluster=w266, "GraphData.Persistent Data.Graph Props.Scale Properties.X.Format"=w265) -> (w270:T15)
            n105 = Build Array(w269) -> (w268:refnum<vi>[])
            n106 = call "XY Set Control Enable State.vi"("error in (no error)"=w264, "Enabled?"=w263, "Controls"=w268) -> ("error out"=w267:errorcluster)  [unwired: 8 in]
          }
          event Value Change {
            n107 = event-data() -> ("NewVal"=w275:T8)  [unwired: 1 in]
            n108 = Bundle By Name(cluster=w276, "GraphData.Persistent Data.Graph Props.Scale Properties.Y.Precision:"=w275) -> (w277:T15)
          }
          event "Y.Label": Value Change {
            n109 = event-data() -> ("NewVal"=w279:string)  [unwired: 1 in]
            n110 = Bundle By Name(cluster=w282, "GraphData.Persistent Data.Graph Props.Scale Properties.Y.Label:"=w279) -> (w280:T15)
          }
          event "Y.Label.Default": Value Change {
            n111 = event-data() -> ("NewVal"=w284:bool)  [unwired: 1 in]
            n112 = Bundle By Name(cluster=w287, "GraphData.Persistent Data.Graph Props.Scale Properties.Y.DefLabel"=w284) -> (w285:T15)
          }
          event "Y.Label.Visible": Value Change {
            n113 = event-data() -> ("NewVal"=w289:bool)  [unwired: 1 in]
            n114 = Bundle By Name(cluster=w292, "GraphData.Persistent Data.Graph Props.Scale Properties.Y.LabelVis"=w289) -> (w290:T15)
          }
          event "Y.Autoscale": Value Change {
            n115 = event-data() -> ("NewVal"=w303:bool)  [unwired: 1 in]
            n116 = Not(x=w303) -> (.not. x?=w302:bool)
            n117 = Unbundle By Name(w307) -> ("GraphData.References.Graph"=w299:refnum<vi>, "References.Y.Max"=w306:refnum<vi>, "References.Y.Min"=w305:refnum<vi>)
            n118 = Bundle By Name(cluster=w307, "GraphData.Persistent Data.Graph Props.Scale Properties.Y.Auto"=w303) -> (w308:T15)
            n119 = Build Array(w306, w305) -> (w300:refnum<vi>[])
            n120 = call "XY Set Control Enable State.vi"("error in (no error)"=w304, "Enabled?"=w302, "Controls"=w300) -> ("error out"=w294:errorcluster)  [unwired: 8 in]
            n121 = property class="XYGraph (strict)"(reference=w299, error in=w294) -> (error out=w298:errorcluster, "YScale.Maximum"=w297:dbl, "YScale.Minimum"=w296:dbl)  [unwired: 1 out]
            n122 = Build Array(w297, w296) -> (w295:dbl[])
            n123 = for {
              shift-right: [w312] -> w301
              shift-left: w298 -> [w313]
              tunnel: w300 -> [w311] mode=indexing
              tunnel: w295 -> [w310] mode=indexing
              n124 = property class="DigNum (strict)"(reference=w311, error in=w313, "Val(Sgnl)"=w310) -> (error out=w312:errorcluster)  [unwired: 1 out]
            }
          }
          event "Y.Max": Value Change {
            n125 = event-data() -> ("NewVal"=w314:dbl)  [unwired: 1 in]
            n126 = Bundle By Name(cluster=w317, "GraphData.Persistent Data.Graph Props.Scale Properties.Y.Max"=w314) -> (w315:T15)
          }
          event "Y.Min": Value Change {
            n127 = event-data() -> ("NewVal"=w319:dbl)  [unwired: 1 in]
            n128 = Bundle By Name(cluster=w322, "GraphData.Persistent Data.Graph Props.Scale Properties.Y.Min"=w319) -> (w320:T15)
          }
          event "X Channel": Value Change {
            n129 = event-data() -> ("NewVal"=w328:i32[])  [unwired: 1 in]
            n130 = Unbundle By Name(w324) -> ("References.X Previous"=w332:refnum<vi>)
            n131 = Empty Array?(array=w328) -> (empty?=w329:bool)
            n132 = Select(t=T18."Disabled and Grayed Out" ("Disabled"), s=w329, f=T18."Enabled" ("Disabled")) -> (s? t:f=w325:T18)
            n133 = property class="Bool"(reference=w332, error in=w331, "DisabledEnum"=w325) -> (error out=w330:errorcluster)  [unwired: 1 out]
          }
          event "Y Channel": Value Change {
            n134 = event-data() -> ("NewVal"=w337:i32[])  [unwired: 1 in]
            n135 = Unbundle By Name(w342) -> ("References.Y Previous"=w341:refnum<vi>)
            n136 = Empty Array?(array=w337) -> (empty?=w338:bool)
            n137 = Select(t=T18."Disabled and Grayed Out" ("Disabled"), s=w338, f=T18."Enabled" ("Disabled")) -> (s? t:f=w334:T18)
            n138 = property class="Bool"(reference=w341, error in=w340, "DisabledEnum"=w334) -> (error out=w339:errorcluster)  [unwired: 1 out]
          }
        }
      }
      frame "Error" {
        n139 = call <vilib>:"Simple Error Handler.vi"("error in (no error)"=w347) -> ()  [unwired: 4 in, 5 out]
      }
      frame "Send Persistent Data" {
        n140 = Unbundle By Name(w356) -> ("GraphData.System.FromDialog"=w354:refnum<user-event>, "GraphData.Persistent Data"=w348:T4)
        n141 = Bundle By Name(cluster=T20 {"DialogMsgType"=enum."Update", "Persistent Data"={"Label"="", "Graph Props"={"Plots"=[], "Legend:Number of Rows"=0, "Scale Properties"={"X.Auto"=FALSE, "X.Min"=0.0, "X.Max"=0.0, "X.IgnoreTS"=FALSE, "X.Precision"=0, "X.Label:"="", "X.LabelVis"=FALSE, "X.DefLabel"=FALSE, "Y.Auto"=FALSE, "Y.Min"=0.0, "Y.Max"=0.0, "Y.Format"=0, "Y.Precision:"=0, "Y.Label:"="", "Y.LabelVis"=FALSE, "Y.DefLabel"=FALSE, "X.Format"=0}, "Legend:Visible"=TRUE, "BgColor"=0, "Last Plot Width"=0, "Resize"=FALSE}, "UDP Data"={"Decimation"=0, "UDP Buffer Size"=0, "History Length"=0.0, "Update Rate"=enum."15 Hz", "Channel Paths"=[], "Channel Names"=[]}}} ("event data"), "DialogMsgType"=XY_Dialog_Msg_Type."Update", "Persistent Data"=w348) -> (w349:T20)
        n142 = Generate User Event(user event=w354, event data cluster=w349, error in=w355) -> (error out=w352:errorcluster)  [unwired: 1 in, 1 out]
      }
      frame "Delete" {
        n143 = Unbundle By Name(w363) -> ("GraphData.System.FromDialog"=w361:refnum<user-event>)
        n144 = Bundle By Name(cluster=T20 {"DialogMsgType"=enum."Update", "Persistent Data"={"Label"="", "Graph Props"={"Plots"=[], "Legend:Number of Rows"=0, "Scale Properties"={"X.Auto"=FALSE, "X.Min"=0.0, "X.Max"=0.0, "X.IgnoreTS"=FALSE, "X.Precision"=0, "X.Label:"="", "X.LabelVis"=FALSE, "X.DefLabel"=FALSE, "Y.Auto"=FALSE, "Y.Min"=0.0, "Y.Max"=0.0, "Y.Format"=0, "Y.Precision:"=0, "Y.Label:"="", "Y.LabelVis"=FALSE, "Y.DefLabel"=FALSE, "X.Format"=0}, "Legend:Visible"=TRUE, "BgColor"=0, "Last Plot Width"=0, "Resize"=FALSE}, "UDP Data"={"Decimation"=0, "UDP Buffer Size"=0, "History Length"=0.0, "Update Rate"=enum."15 Hz", "Channel Paths"=[], "Channel Names"=[]}}} ("event data"), "DialogMsgType"=XY_Dialog_Msg_Type."Delete") -> (w358:T20)
        n145 = Build Array (concatenate)("MACRO - Shut Down", w366) -> (w365:string[])
        n146 = Generate User Event(user event=w361, event data cluster=w358, error in=w362) -> (error out=w359:errorcluster)  [unwired: 1 in, 1 out]
      }
      frame "<------------------ Shut Down ------------------>" {
      }
      frame "Exit" {
        n147 = local write "Tab Control"(enum32{"General", "Format & Precision"}."General" ("Tab Control")) -> ()
      }
      frame "<------------------ Macros ------------------>" {
      }
      frame "MACRO - Initialize" {
        n148 = Build Array (concatenate)(string[] ["Get Control References", "Clear Listbox", "Update FP With Persistent Data"], w380) -> (w379:string[])
      }
      frame "MACRO - Shut Down" {
        n149 = Build Array (concatenate)(string[] ["Exit"], w386) -> (w385:string[])
      }
      frame "MACRO - Send Update & Shut Down" {
        n150 = Build Array (concatenate)(string[] ["Send Persistent Data", "MACRO - Shut Down"], w390) -> (w389:string[])
      }
      frame "<------------------ Initialization ------------------>" {
      }
      frame "Get Control References" {
        n151 = control-ref of="Y Channel"() -> (w405:refnum<vi>)
        n152 = control-ref of="X Channel"() -> (w404:refnum<vi>)
        n153 = control-ref of="Tree Browser"() -> (w406:refnum<vi>)
        n154 = control-ref of="Plot Area Background Color"() -> (w407:refnum<vi>)
        n155 = control-ref of="Y Next"() -> (w401:refnum<vi>)
        n156 = control-ref of="X Previous"() -> (w400:refnum<vi>)
        n157 = control-ref of="Y Previous"() -> (w399:refnum<vi>)
        n158 = control-ref of="X Next"() -> (w402:refnum<vi>)
        n159 = control-ref of="X.Label.Default"() -> (w420:refnum<vi>)
        n160 = control-ref of="X.Label.Visible"() -> (w419:refnum<vi>)
        n161 = control-ref of="X.Autoscale"() -> (w418:refnum<vi>)
        n162 = control-ref of="Y.Label.Default"() -> (w412:refnum<vi>)
        n163 = control-ref of="Y.Label.Visible"() -> (w411:refnum<vi>)
        n164 = control-ref of="Y.Autoscale"() -> (w410:refnum<vi>)
        n165 = control-ref of="Decimation:"() -> (w398:refnum<vi>)
        n166 = control-ref of="UDP Buffer Size:"() -> (w396:refnum<vi>)
        n167 = control-ref of="History Length:"() -> (w397:refnum<vi>)
        n168 = control-ref of="X.Max"() -> (w417:refnum<vi>)
        n169 = control-ref of="X.Min"() -> (w416:refnum<vi>)
        n170 = control-ref of="Y.Max"() -> (w409:refnum<vi>)
        n171 = control-ref of="Y.Min"() -> (w408:refnum<vi>)
        n172 = control-ref of="Graph Title"() -> (w423:refnum<vi>)
        n173 = control-ref of="X.Label"() -> (w421:refnum<vi>)
        n174 = control-ref of="Y.Label"() -> (w413:refnum<vi>)
        n175 = control-ref of="X.Format"() -> (w403:refnum<vi>)
        n176 = control-ref of="X.Precision"() -> (w422:refnum<vi>)
        n177 = control-ref of="Y.Format"() -> (w415:refnum<vi>)
        n178 = control-ref of="Y.Precision"() -> (w414:refnum<vi>)
        n179 = Bundle By Name(cluster=w427, "References.BgColor"=w407, "References.Title"=w423, "References.X.Precision"=w422, "References.X.Label"=w421, "References.X.Label.Default"=w420, "References.X.Label.Visible"=w419, "References.X.Autoscale"=w418, "References.X.Max"=w417, "References.X.Min"=w416, "References.Y.Format"=w415, "References.Y.Precision"=w414, "References.Y.Label"=w413, "References.Y.Label.Default"=w412, "References.Y.Label.Visible"=w411, "References.Y.Autoscale"=w410, "References.Y.Max"=w409, "References.Y.Min"=w408, "References.Alias TreeBrowser"=w406, "References.X Channel Listbox"=w404, "References.Y Channel Listbox"=w405, "References.X.Format"=w403, "References.X Next"=w402, "References.Y Next"=w401, "References.X Previous"=w400, "References.Y Previous"=w399, "References.Decimation"=w398, "References.UDP Buffer Size"=w396, "References.History Length"=w397) -> (w426:T15)
      }
      frame "Update FP With Persistent Data" {
        # "Only happens at start up so the FP controls and indiators are initialized"
        n180 = Unbundle By Name(w436) -> ("GraphData.System.Root"=w437:refnum<k24>, "GraphData.Persistent Data"=w429:T4, "References"=w438:T16)
        n181 = Unbundle By Name(w429) -> ("UDP Data.Update Rate"=w428:T11)
        n182 = call "XY Dialog - Update FP Settings With Persistent Data.vi"("GraphData.System.Root"=w437, "error in (no error)"=w440, "References"=w438, "Persistent Data"=w429) -> ("error out"=w431:errorcluster)  [unwired: 7 in]
        n183 = control-ref of="Update Rate:"() -> (w432:refnum<vi>)
        n184 = property class="Enum (strict)"(reference=w432, error in=w431, "Val(Sgnl)"=w428) -> (error out=w430:errorcluster)  [unwired: 1 out]
        n185 = call "XY Dialog - Initialize Tree.vi"("error in (no error)"=w430, "TreeAliasBrowserWF"=w433, "GraphData.System.Root"=w437) -> ("error out"=w439:errorcluster, "Event Registration Refnum"=w435:refnum<event-registration>)  [unwired: 7 in]
        n186 = Bundle By Name(cluster=w436, "GraphData.System.TreeBrowserEventReg"=w435) -> (w434:T15)
      }
      frame "Clear Listbox" {
        w442 = i32[] [] ("Value (Signaling)")
        w443 = string[][] [] ("Item Names")
        n187 = Unbundle By Name(w449) -> ("References.Y Channel Listbox"=w445:refnum<vi>, "References.X Channel Listbox"=w447:refnum<vi>)
        n188 = property class="MCListbox (strict)"(reference=w447, error in=w448, "ItemNames"=w443, "Val(Sgnl)"=w442) -> (error out=w446:errorcluster)  [unwired: 1 out]
        n189 = property class="MCListbox (strict)"(reference=w445, error in=w446, "ItemNames"=w443, "Val(Sgnl)"=w442) -> (error out=w444:errorcluster)  [unwired: 1 out]
      }
    }
    n190 = Unbundle By Name(w11) -> ("GraphData.System.ErrFlag"=w10:bool)
    n191 = Compound Arithmetic op=AND(invert w10, w8) -> (w9:bool)
    n192 = case shown="False" w9 {
      selector: w9 -> [_ w24]
      tunnel: w18 -> [w23 w27]
      tunnel: [w23 w28] -> w16
      tunnel: [w22 w25] -> w12
      tunnel: w11 -> [w22 w26]
      frame False {
      }
      frame True {
        n193 = Bundle By Name(cluster=w26, "GraphData.System.ErrFlag"=w24) -> (w25:T15)
        n194 = Build Array (concatenate)("Error", w27) -> (w28:string[])
      }
    }
  }
